vi "CLC_JIO_Recode_ALL.vi"(4 "error in":errorcluster, 5 "Mode":enum16{"Standy", "Tx", "Rx"}(ring)=enum."Tx", 6 "FileName":string="SingleCh_", 7 "Function":T1, 8 "ele_att":i32=255, 9 "com_att":i32=255, 10 "UD_att":i32=255, 11 "pol":u16) -> (0 "error out":errorcluster, 3 "standard output":string)   [LabVIEW 2023, in "CLC_JIO_FTDI.lvlib"]
uses:
  CTL/JIO_FPGA_FTDI.ctl
  CLC_JIO_FTDI.lvlib
panel:
  out "standard error":string
  out "floder?":bool
  # "0:H\n1:V\n2:H+V"
  # "0-15"
  # "0-15"
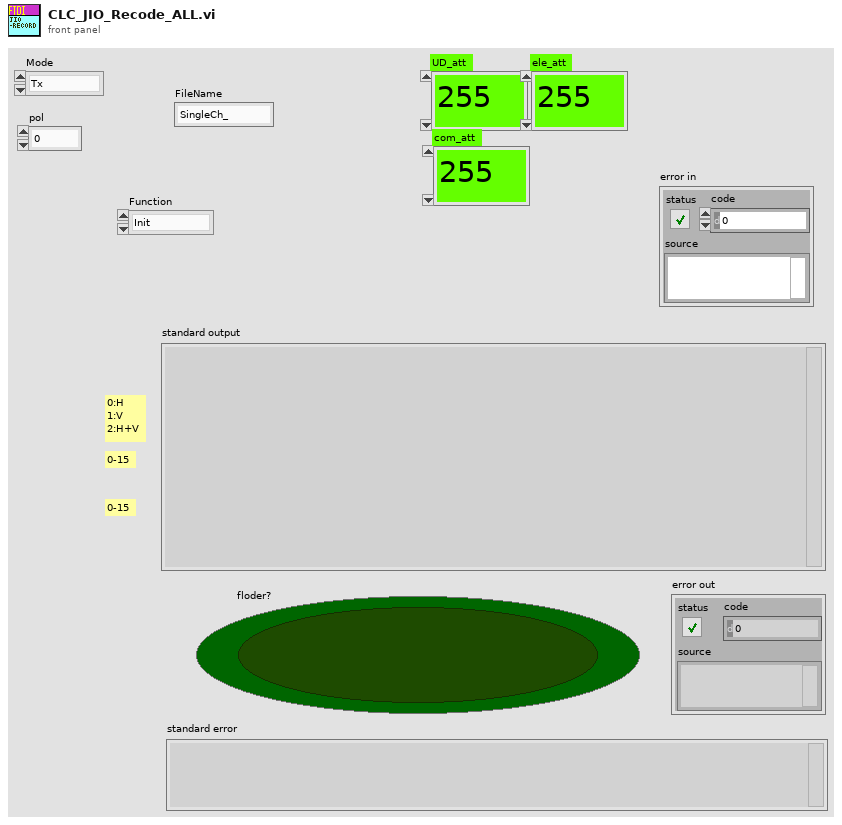
[diagram p1: front panel]
types:
  T1 = typedef "JIO_FPGA_FTDI.ctl" = enum16{"Init", "Close", "UD", "BFIC"}
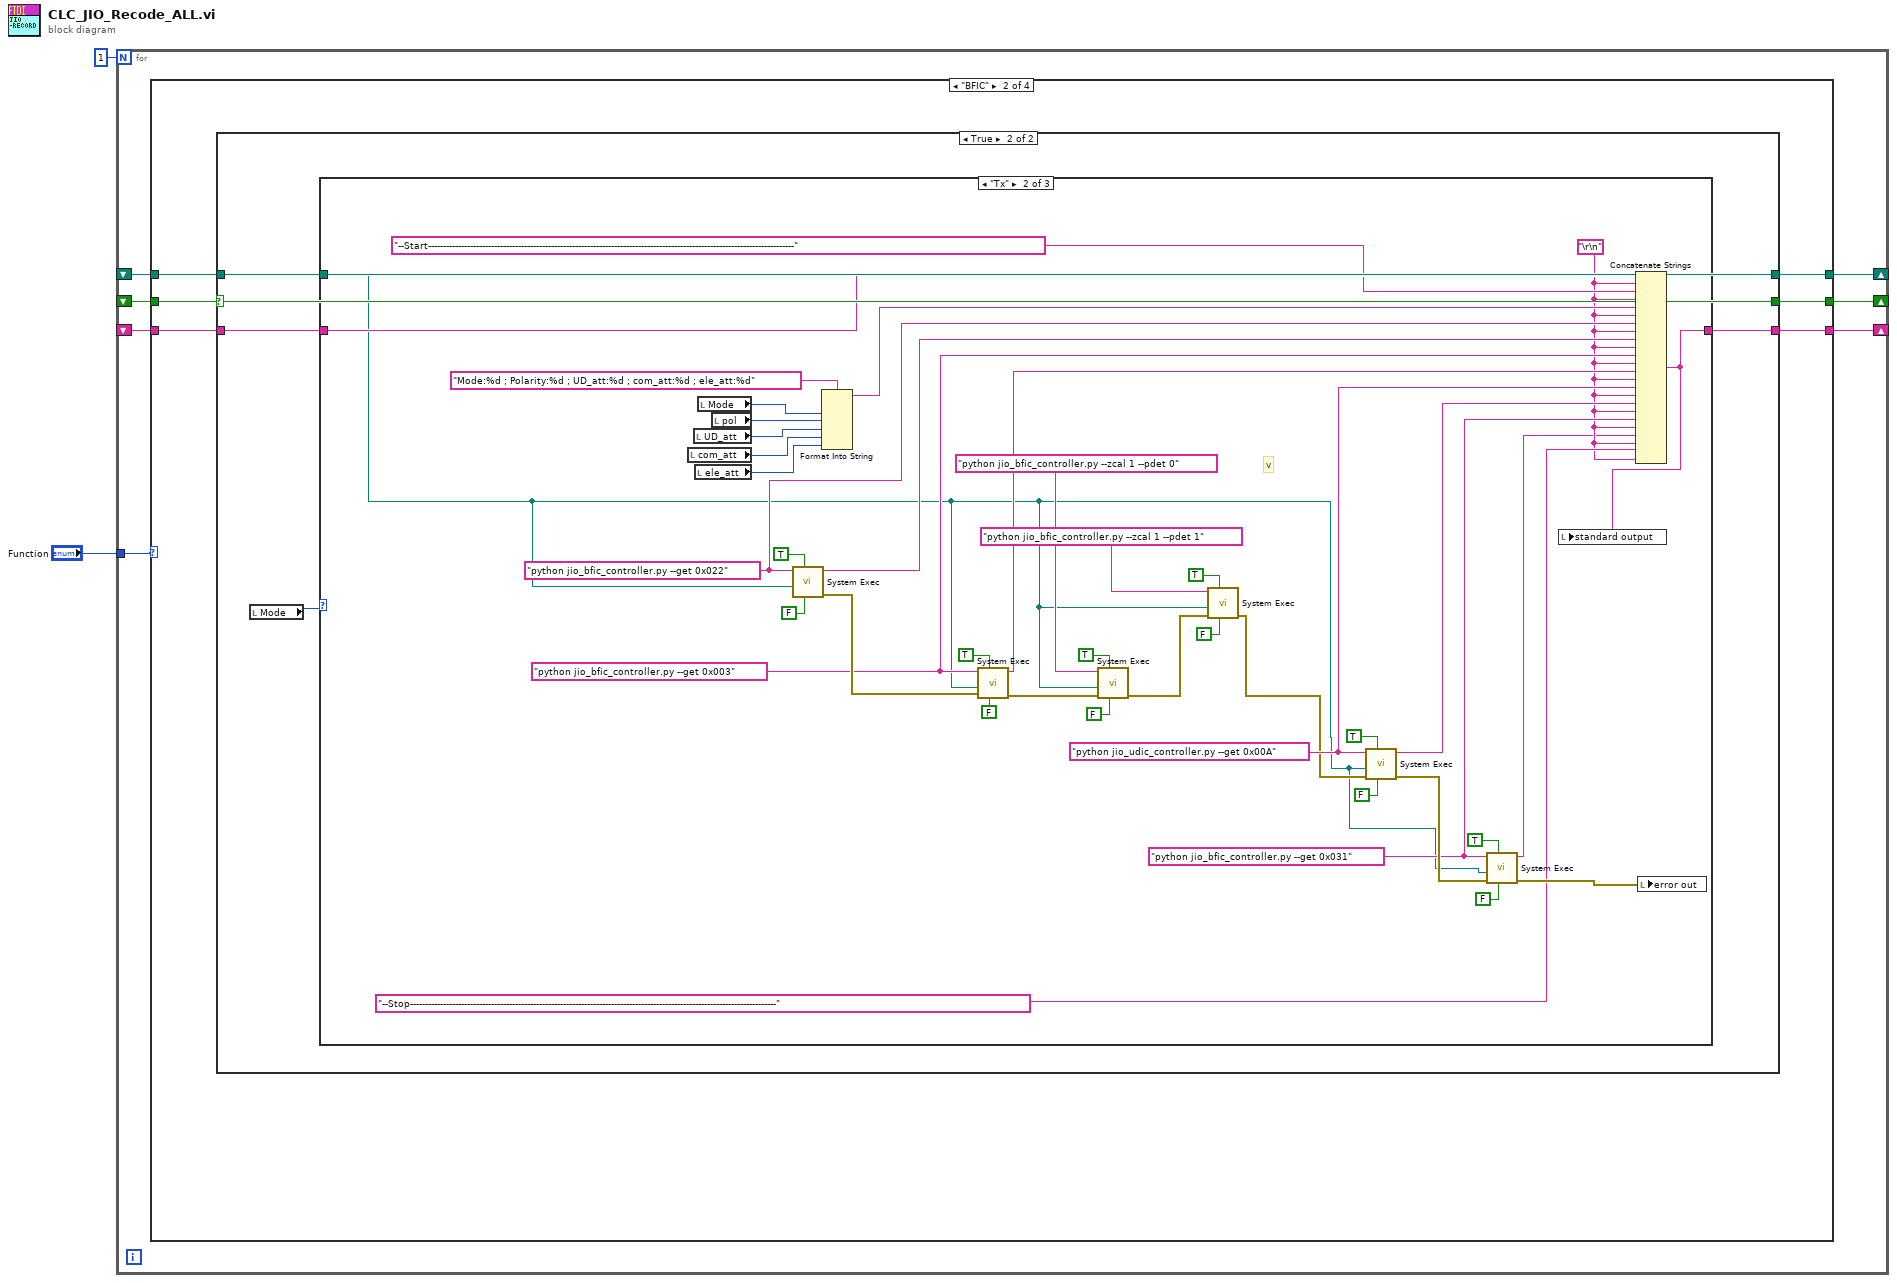
[diagram p0: block diagram]
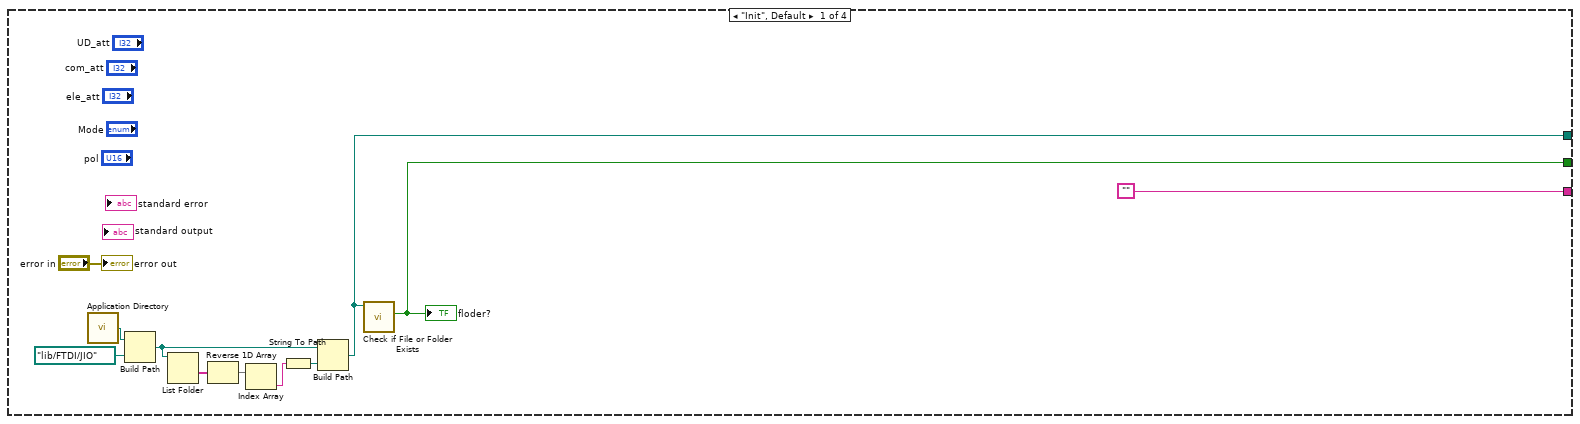
[diagram p2: hidden frame]
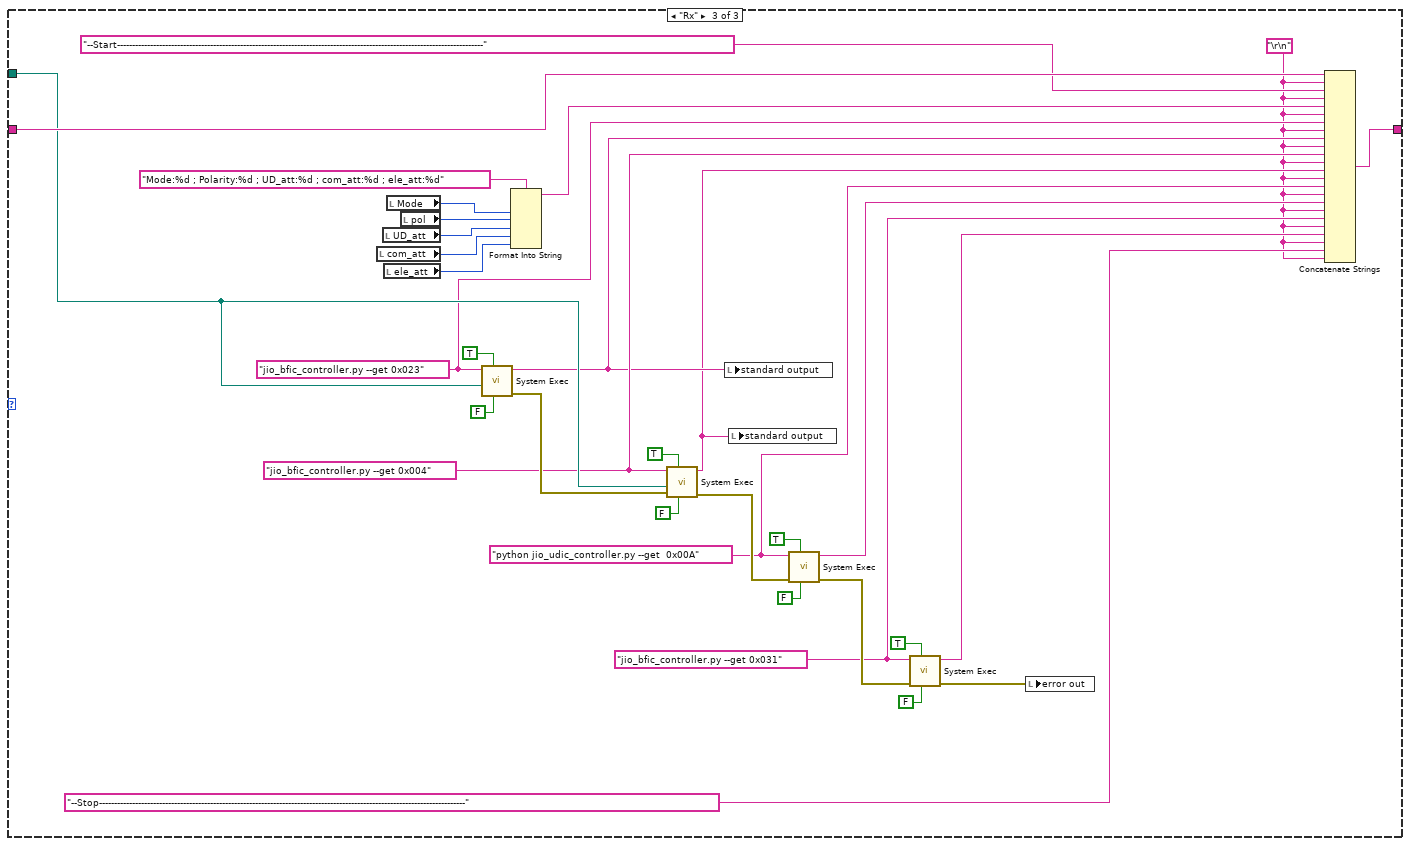
[diagram p5: hidden frame]
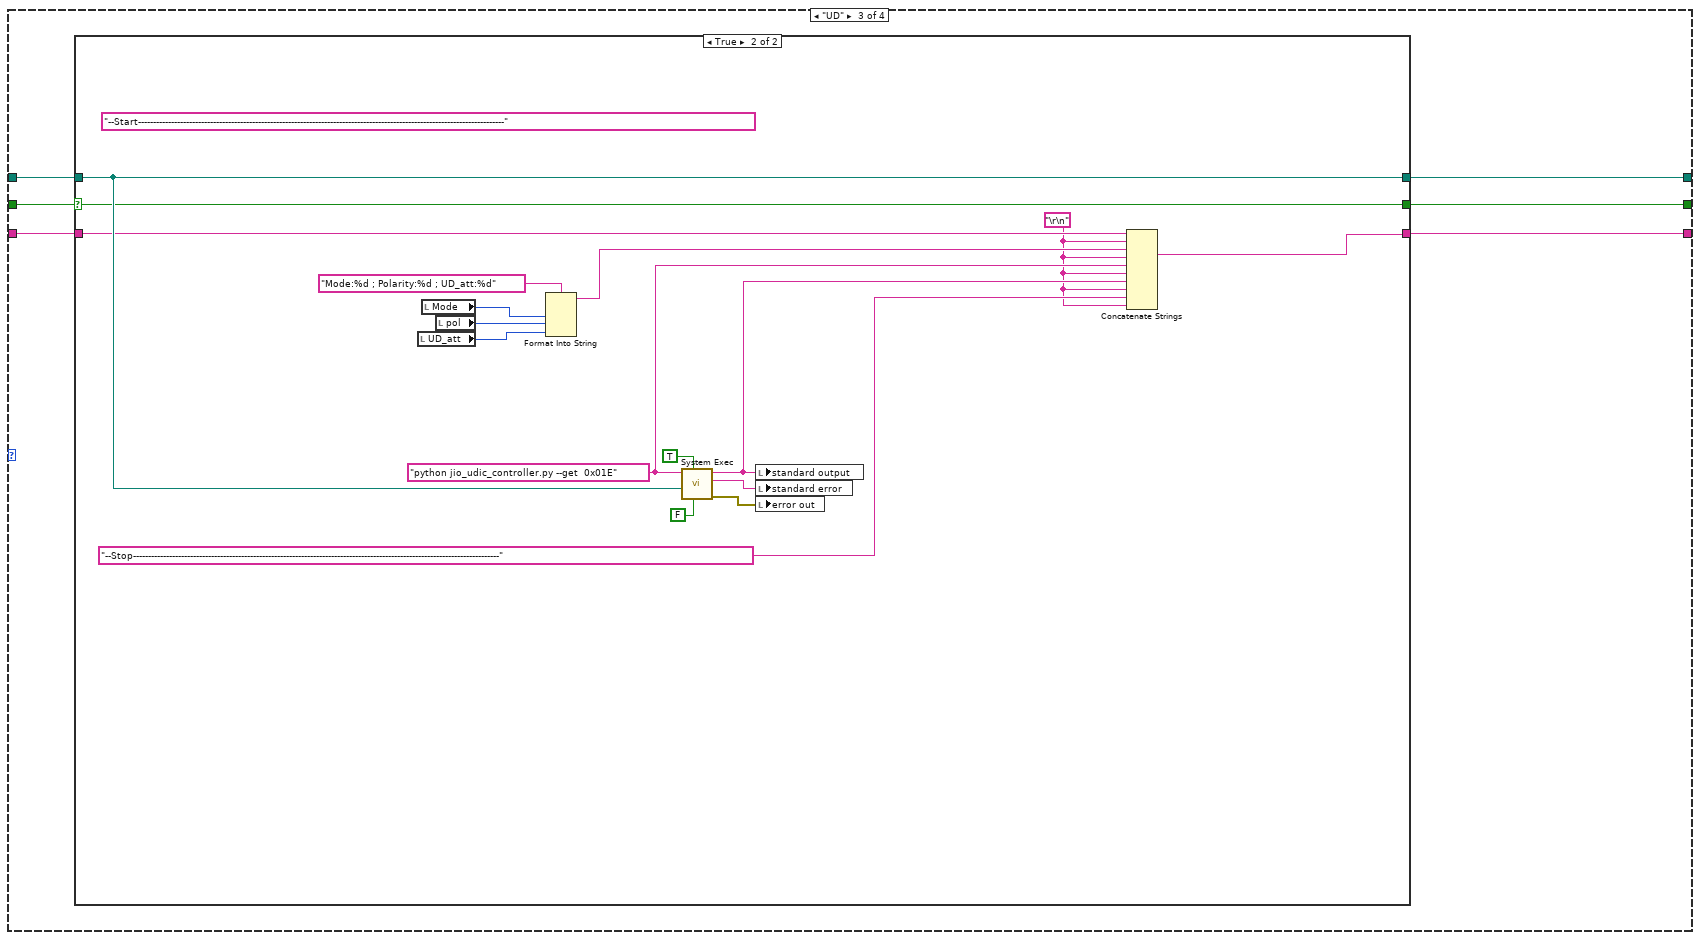
[diagram p6: hidden frame]
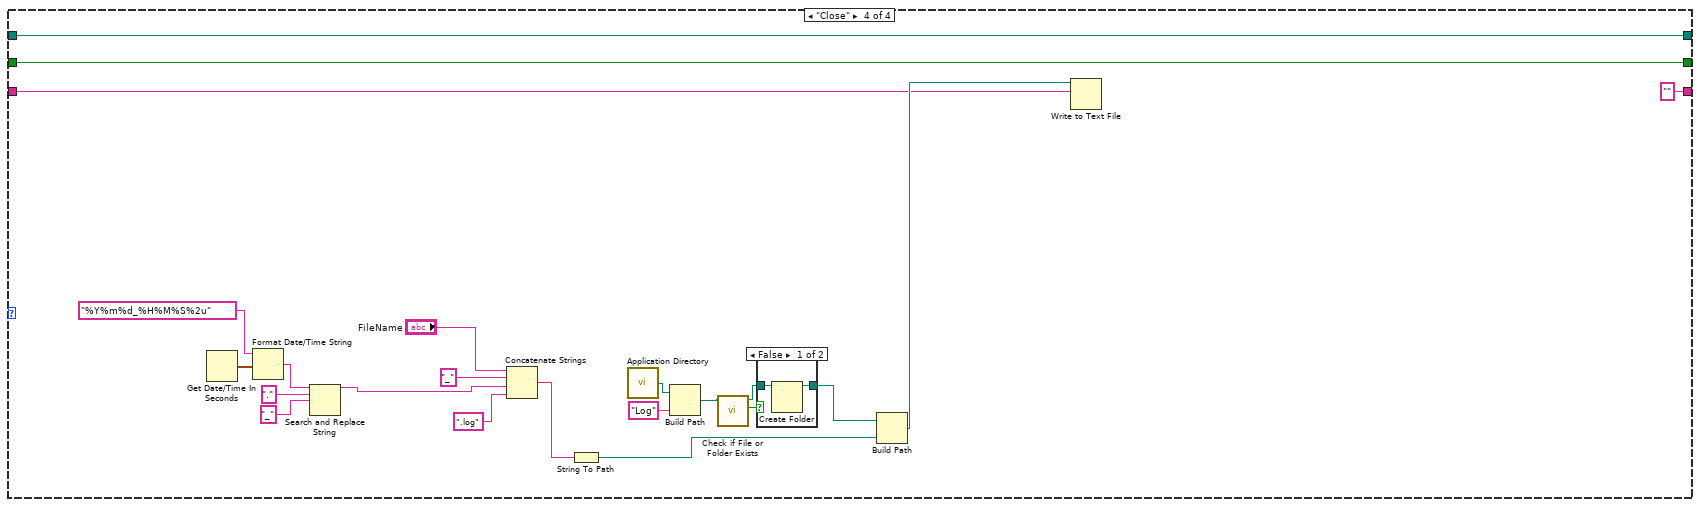
[diagram p8: hidden frame]
diagram:
  n1 = for {
    N: 1 -> [_]
    tunnel: "Function" -> [w9]
    shift-right: [w8] -> _
    shift-left: _ -> [w4]
    shift-right: [w7] -> _
    shift-left: _ -> [w5]
    shift-right: [w6] -> _
    shift-left: _ -> [w3]
    n2 = case shown="\"BFIC\"" w9 {
      tunnel: [w13 w24 w113 w136] -> w8
      tunnel: [w12 w23 w112 w137] -> w7
      tunnel: ["" w22 w111 ""] -> w6
      tunnel: w5 -> [_ w26 w115 w137]
      tunnel: w4 -> [_ w25 w114 w136]
      tunnel: w3 -> [_ w21 w110 w139]
      frame "Init", Default {
        n3 = call <vilib>:"Application Directory.vi"() -> ("Application Directory"=w19:path)
        n4 = Build Path(base path=w19, name or relative path=path "lib/FTDI/JIO") -> (appended path=w20:path)
        n5 = List Folder(path=w20) -> (folder names=w15:string[])  [unwired: 3 in, 3 out]
        n6 = Reverse 1D Array(array=w15) -> (reversed array=w16:string[])
        n7 = Index Array(array=w16) -> (element=w17:string)  [unwired: 1 in]
        n8 = String To Path(string=w17) -> (path=w18:path)
        n9 = Build Path(base path=w20, name or relative path=w18) -> (appended path=w13:path)
        n10 = call <vilib>:"Check if File or Folder Exists.vi"("path"=w13) -> ("file or folder exists?"=w12:bool)  [unwired: 8 in, 2 out]
        "floder?" <- w12
        "error out" <- "error in"
      }
      frame "BFIC" {
        n11 = case shown="True" w26 {
          selector: w26 -> [w28 w33]
          tunnel: w25 -> [w29 w34]
          tunnel: [w29 w34] -> w24
          tunnel: [w28 w33] -> w23
          tunnel: [w27 w31] -> w22
          tunnel: w21 -> [w27 w32]
          frame False {
          }
          frame True {
            n12 = local read "Mode"() -> (w30:enum16{"Standy", "Tx", "Rx"})
            n13 = case shown="\"Tx\"" w30 {
              tunnel: w34 -> [_ w36 w100]
              tunnel: w32 -> [w35 w74 w107]
              tunnel: [w35 w46 w106] -> w31
              frame "Standy", Default {
              }
              frame "Tx" {
                w52 = "python jio_udic_controller.py --get 0x00A" ("string")
                w50 = "python jio_bfic_controller.py --get 0x031" ("string")
                w48 = "\r\n"
                w61 = "python jio_bfic_controller.py --get 0x003" ("string")
                w64 = "python jio_bfic_controller.py --get 0x022" ("string")
                # "v"
                n14 = local read "com_att"() -> (w68:i32)
                n15 = local read "UD_att"() -> (w71:i32)
                n16 = local read "ele_att"() -> (w67:i32)
                n17 = local read "Mode"() -> (w73:enum16{"Standy", "Tx", "Rx"})
                n18 = local read "pol"() -> (w72:u16)
                n19 = call <vilib>:"System Exec.vi"("run minimized? (F)"=FALSE, "wait until completion? (T)"=TRUE, "working directory"=w36, "command line"=w64) -> ("error out"=w66:errorcluster, "standard output"=w60:string)  [unwired: 4 in, 2 out]
                n20 = Format Into String(format string="Mode:%d ; Polarity:%d ; UD_att:%d ; com_att:%d ; ele_att:%d" ("string"), w73, w72, w71, w68, w67) -> (resulting string=w62:string)  [unwired: 2 in, 1 out]
                n21 = call <vilib>:"System Exec.vi"("run minimized? (F)"=FALSE, "wait until completion? (T)"=TRUE, "error in (no error)"=w66, "working directory"=w36, "command line"=w61) -> ("error out"=w41:errorcluster, "standard output"=w59:string)  [unwired: 3 in, 2 out]
                n22 = call <vilib>:"System Exec.vi"("run minimized? (F)"=FALSE, "wait until completion? (T)"=TRUE, "error in (no error)"=w41, "working directory"=w36, "command line"="python jio_bfic_controller.py --zcal 1 --pdet 0" ("string")) -> ("error out"=w39:errorcluster)  [unwired: 3 in, 3 out]
                n23 = call <vilib>:"System Exec.vi"("run minimized? (F)"=FALSE, "wait until completion? (T)"=TRUE, "error in (no error)"=w39, "working directory"=w36, "command line"="python jio_bfic_controller.py --zcal 1 --pdet 1" ("string")) -> ("error out"=w40:errorcluster)  [unwired: 3 in, 3 out]
                n24 = call <vilib>:"System Exec.vi"("run minimized? (F)"=FALSE, "wait until completion? (T)"=TRUE, "error in (no error)"=w40, "working directory"=w36, "command line"=w52) -> ("error out"=w54:errorcluster, "standard output"=w51:string)  [unwired: 3 in, 2 out]
                n25 = call <vilib>:"System Exec.vi"("run minimized? (F)"=FALSE, "wait until completion? (T)"=TRUE, "error in (no error)"=w54, "working directory"=w36, "command line"=w50) -> ("error out"=w53:errorcluster, "standard output"=w47:string)  [unwired: 3 in, 2 out]
                n26 = Concatenate Strings(w74, w48, "--Start--------------------------------------------------------------------------------------------------------------------------" ("string"), w48, w62, w48, w64, w48, w60, w48, w61, w48, w59, w48, w52, w48, w51, w48, w50, w48, w47, w48, "--Stop--------------------------------------------------------------------------------------------------------------------------" ("string"), w48) -> (w46:string)
                n27 = local write "standard output"(w46) -> ()
                n28 = local write "error out"(w53) -> ()
              }
              frame "Rx" {
                w82 = "python jio_udic_controller.py --get  0x00A" ("string")
                w80 = "jio_bfic_controller.py --get 0x031" ("string")
                w77 = "\r\n"
                w92 = "jio_bfic_controller.py --get 0x004" ("string")
                w95 = "jio_bfic_controller.py --get 0x023" ("string")
                n29 = local read "com_att"() -> (w99:i32)
                n30 = local read "UD_att"() -> (w103:i32)
                n31 = local read "ele_att"() -> (w98:i32)
                n32 = local read "Mode"() -> (w105:enum16{"Standy", "Tx", "Rx"})
                n33 = local read "pol"() -> (w104:u16)
                n34 = call <vilib>:"System Exec.vi"("run minimized? (F)"=FALSE, "wait until completion? (T)"=TRUE, "working directory"=w100, "command line"=w95) -> ("error out"=w97:errorcluster, "standard output"=w91:string)  [unwired: 4 in, 2 out]
                n35 = Format Into String(format string="Mode:%d ; Polarity:%d ; UD_att:%d ; com_att:%d ; ele_att:%d" ("string"), w105, w104, w103, w99, w98) -> (resulting string=w93:string)  [unwired: 2 in, 1 out]
                n36 = call <vilib>:"System Exec.vi"("run minimized? (F)"=FALSE, "wait until completion? (T)"=TRUE, "error in (no error)"=w97, "working directory"=w100, "command line"=w92) -> ("error out"=w85:errorcluster, "standard output"=w90:string)  [unwired: 3 in, 2 out]
                n37 = local write "standard output"(w91) -> ()
                n38 = local write "standard output"(w90) -> ()
                n39 = call <vilib>:"System Exec.vi"("run minimized? (F)"=FALSE, "wait until completion? (T)"=TRUE, "error in (no error)"=w85, "command line"=w82) -> ("error out"=w84:errorcluster, "standard output"=w81:string)  [unwired: 4 in, 2 out]
                n40 = call <vilib>:"System Exec.vi"("run minimized? (F)"=FALSE, "wait until completion? (T)"=TRUE, "error in (no error)"=w84, "command line"=w80) -> ("error out"=w83:errorcluster, "standard output"=w79:string)  [unwired: 4 in, 2 out]
                n41 = local write "error out"(w83) -> ()
                n42 = Concatenate Strings(w107, w77, "--Start--------------------------------------------------------------------------------------------------------------------------" ("string"), w77, w93, w77, w95, w77, w91, w77, w92, w77, w90, w77, w82, w77, w81, w77, w80, w77, w79, w77, "--Stop--------------------------------------------------------------------------------------------------------------------------" ("string"), w77) -> (w106:string)
              }
            }
          }
        }
      }
      frame "UD" {
        n43 = case shown="True" w115 {
          selector: w115 -> [w117 w130]
          tunnel: w114 -> [w118 w131]
          tunnel: [w118 w131] -> w113
          tunnel: [w117 w130] -> w112
          tunnel: [w116 w127] -> w111
          tunnel: w110 -> [w116 w129]
          frame False {
          }
          frame True {
            w119 = "\r\n"
            (unwired) "--Start--------------------------------------------------------------------------------------------------------------------------" ("string")
            w122 = "python jio_udic_controller.py --get  0x01E" ("string")
            n44 = local read "UD_att"() -> (w124:i32)
            n45 = local read "Mode"() -> (w126:enum16{"Standy", "Tx", "Rx"})
            n46 = local read "pol"() -> (w125:u16)
            n47 = Format Into String(format string="Mode:%d ; Polarity:%d ; UD_att:%d" ("string"), w126, w125, w124) -> (resulting string=w123:string)  [unwired: 2 in, 1 out]
            n48 = call <vilib>:"System Exec.vi"("run minimized? (F)"=FALSE, "wait until completion? (T)"=TRUE, "working directory"=w131, "command line"=w122) -> ("error out"=w132:errorcluster, "standard error"=w133:string, "standard output"=w121:string)  [unwired: 4 in, 1 out]
            n49 = local write "standard output"(w121) -> ()
            n50 = local write "standard error"(w133) -> ()
            n51 = local write "error out"(w132) -> ()
            n52 = Concatenate Strings(w129, w119, w123, w119, w122, w119, w121, w119, "--Stop--------------------------------------------------------------------------------------------------------------------------" ("string"), w119) -> (w127:string)
          }
        }
      }
      frame "Close" {
        n53 = Get Date/Time In Seconds() -> (seconds since 1Jan1904=w152:timestamp)
        n54 = Format Date/Time String(time format string (%c)="%Y%m%d_%H%M%S%2u", seconds (now)=w152) -> (date/time string=w150:string)  [unwired: 1 in]
        n55 = Search and Replace String(input string=w150, search string=".", replace string="_") -> (result string=w147:string)  [unwired: 5 in, 3 out]
        n56 = Concatenate Strings("FileName", "_" ("delimiter (\\t)"), w147, ".log" ("delimiter (\\t)")) -> (w155:string)
        n57 = String To Path(string=w155) -> (path=w156:path)
        n58 = call <vilib>:"Application Directory.vi"() -> ("Application Directory"=w154:path)
        n59 = Build Path(base path=w154, name or relative path="Log") -> (appended path=w144:path)
        n60 = call <vilib>:"Check if File or Folder Exists.vi"("path"=w144) -> ("file or folder exists?"=w146:bool, "dup path"=w145:path)  [unwired: 8 in, 1 out]
        n61 = case shown="False" w146 {
          tunnel: w145 -> [w159 w160]
          tunnel: [w158 w160] -> w143
          frame False {
            n62 = Create Folder(path (use dialog)=w159) -> (created path=w158:path)  [unwired: 2 in, 2 out]
          }
          frame True {
          }
        }
        n63 = Build Path(base path=w143, name or relative path=w156) -> (appended path=w142:path)
        n64 = Write to Text File(file (use dialog)=w142, text=w139) -> ()  [unwired: 2 in, 3 out]
      }
    }
  }
